vi "Measurement Data Convert (Harmonics).vi"(8 "error in (no error)":errorcluster, 9 "Item Number Offset (1)":i32=1 min=1 max=64, 10 "Measurement Data (Empty)":string, 11 "VISA resource name":refnum<visa-resource-name>) -> (0 "error out":errorcluster, 1 "Measurement":dbl[][](array[numeric]), 2 "Function":string[](array[string]), 3 "VISA resource name out":refnum<visa-resource-name>)   [LabVIEW 2021, in "Yokogawa WT1800 Series.lvlib"]
doc: "Transforms measurement datas into harmonics numeric data list values."
uses:
  <instrlib>/Yokogawa WT1800 Series/Yokogawa WT1800 Series.lvlib
  <instrlib>/Yokogawa WT1800 Series/Public/Action-Status/Query Numeric (Harmonics).vi
panel:
  # "Total        DC            1             2              3             4"
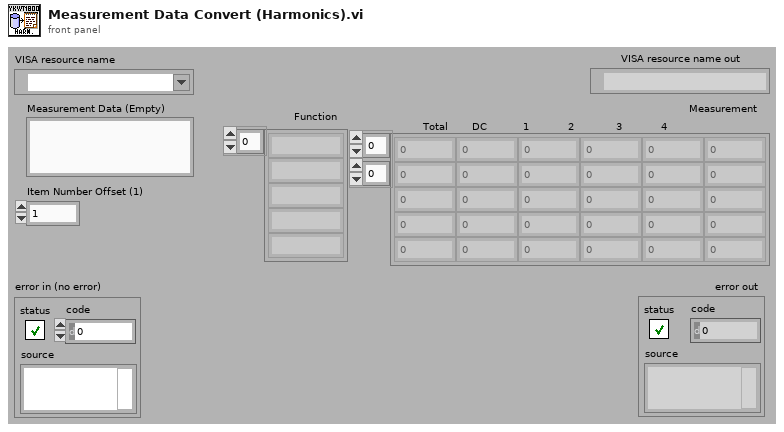
[diagram p1: front panel]
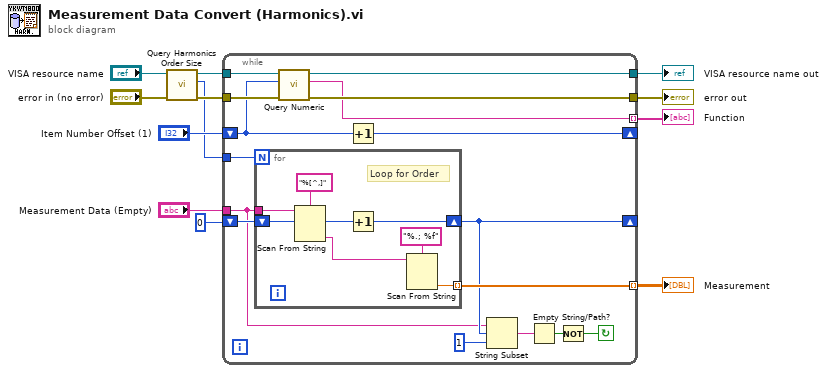
[diagram p0: block diagram]
diagram:
  n1 = call <instrlib>:"Query Harmonics Order Size.vi"("error in (no error)"="error in (no error)", "VISA resource name"="VISA resource name") -> ("error out"=w3:errorcluster, "Number of Harmonics Order"=w2:i32, "VISA resource name out"=w4:refnum<visa-resource-name>)  [unwired: 7 in]
  n2 = while {
    tunnel: [w27] -> w1 mode=indexing
    tunnel: "Measurement Data (Empty)" -> [w13]
    shift-right: [w14] -> _
    shift-left: 0 -> [w28]
    tunnel: w4 -> [w26]
    tunnel: w3 -> [w25]
    shift-right: [w23] -> _
    shift-left: "Item Number Offset (1)" -> [w24]
    tunnel: [w22] -> w9
    tunnel: [w21] -> w8
    tunnel: [w20] -> w7 mode=indexing
    tunnel: w2 -> [w19]
    stop <- w15 continue-if-true
    n3 = for {
      N: w19 -> [_]
      tunnel: w13 -> [w29]
      tunnel: [w32] -> w27 mode=indexing
      shift-right: [w30] -> w14
      shift-left: w28 -> [w35]
      # "Loop for Order"
      n4 = Scan From String(format string="%[^,]", input string=w29, initial scan location=w35) -> (offset past scan=w34:u32, output 1=w33:string)  [unwired: 2 in, 2 out]
      n5 = Increment(x=w34) -> (x+1=w30:u32)
      n6 = Scan From String(format string="%.; %f" ("形式文字列"), input string=w33) -> (output 1=w32:dbl)  [unwired: 3 in, 3 out]
    }
    n7 = call-poly <instrlib>:"Query Numeric.vi"("error in (no error)"=w25, "Item (1)"=w24, "VISA resource name"=w26) -> ("error out"=w21:errorcluster, "Function"=w20:string, "VISA resource name out"=w22:refnum<visa-resource-name>)  [unwired: 6 in]
    n8 = Increment(x=w24) -> (x+1=w23:i32)
    n9 = String Subset(string=w13, offset (0)=w14, length (rest)=1) -> (substring=w17:string)
    n10 = Empty String/Path?(string/path=w17) -> (empty?=w18:bool)
    n11 = Not(x=w18) -> (.not. x?=w15:bool)
  }
  "error out" <- w8
  "VISA resource name out" <- w9
  "Measurement" <- w1
  "Function" <- w7
